vi "sCRIPT Bckup.vi"   [LabVIEW 2020]
uses:
  <userlib>/_OpenG.lib/lvzip/lvzip.llb/ZLIB Open ZIP Mode__ogtk.ctl
  <vilib>/addons/database/Connection.llb/Conn Execute.vi
  <vilib>/addons/database/Recordset.llb/Rec Fetch Recordset Data (R).vi
  <vilib>/addons/database/Recordset.llb/Rec Destroy - Connection.vi
  MS SQL/MS_Global.vi
  <vilib>/addons/database/NI_Database_API.lvlib
types:
  T1 = typedef "ZLIB Open ZIP Mode__ogtk.ctl" = enum16{"create new", "append to end", "append to archive"}
  T2 = typedef "TD SQL.ctl" = cluster{"MS SQL Connection":T3, "UDL File":path, "Time":string, "DCODE":string, "WIP+1":i64, "MC No?":i32, "POKAYOKE?":bool, "Expected Result":string, "Result [Status]":string, "Clock":dbl, "RFID":string, "WIP Queue":refnum<queue>, "TS Parameter":T4, "Data_Queue":refnum<queue>[], "RFID Serial No.":string}
  T3 = typedef "NI_Database_API.lvlib/Conn ObjectReference.ctl" = refnum<k1>
  T4 = typedef "TS_Parameter.ctl" = cluster{"ProfitCenterCode":string, "LineCode":string, "WorkOrderNumber":string, "Model":string, "Model_with_Prefix":string, "VendorCode":string, "SetParameterDateCode":string, "PokaYoke":i32, "Target":i32, "Live_DateCode":string, "CustomerPartNumber":string, "Hand":string, "sBarcode":bool, "FCA":i32, "Ent_Stamp":timestamp, "STS_CD":dbl}
  T5 = cluster{"Data Path":path, "Calibration Path":path, "Settings Path":path, "Script Path":path, "DAQ Support":path, "Reporting Desktop":path, "Help":path}
  T6 = typedef "NI_Database_API.lvlib/Rec ObjectReference.ctl" = refnum<k1>
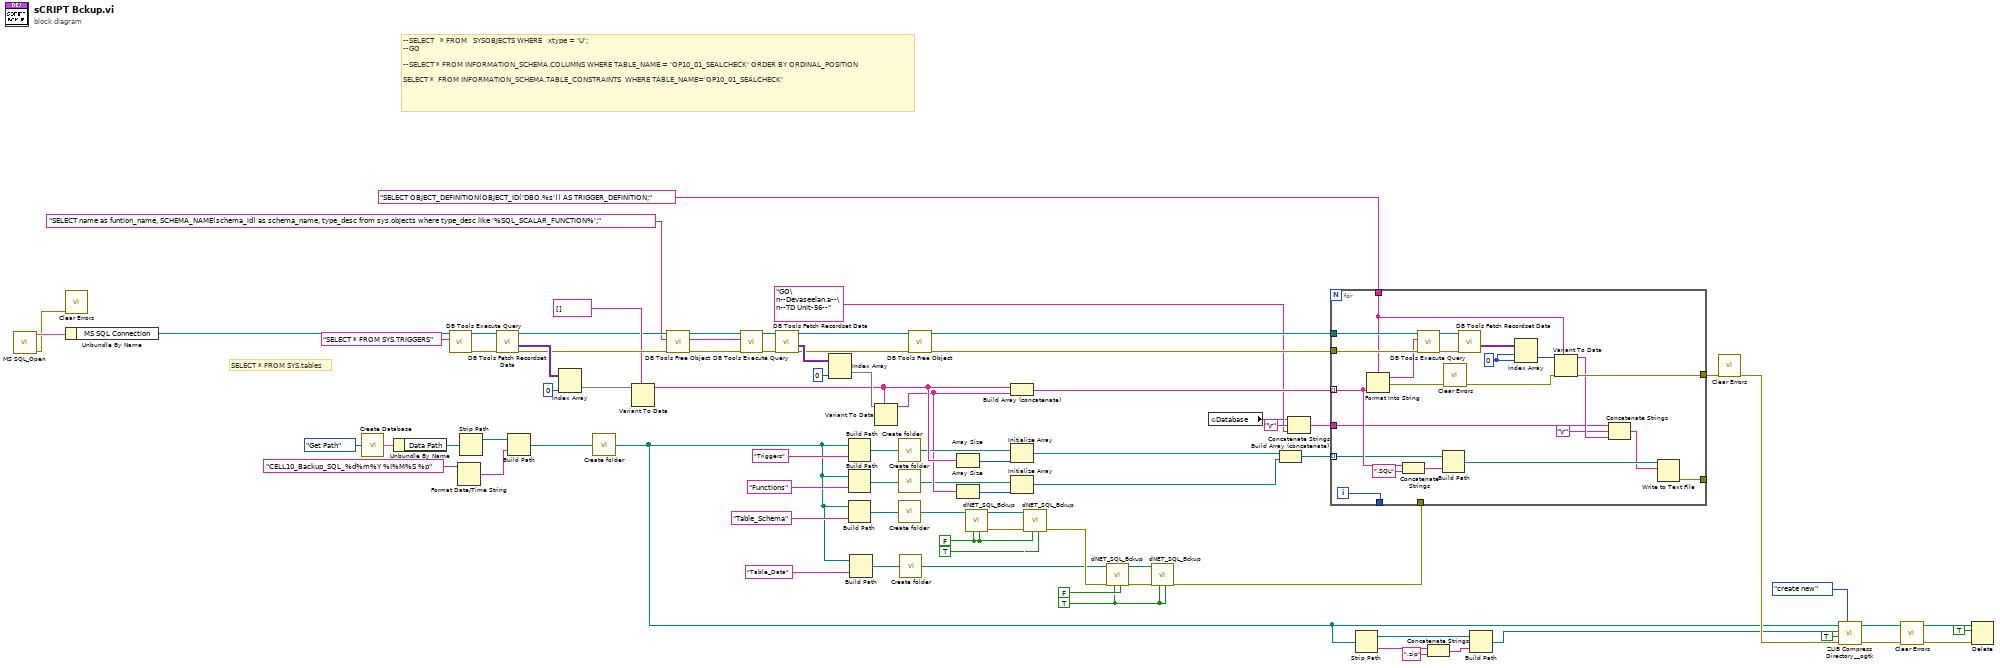
[diagram p0: block diagram]
diagram:
  w2 = TRUE ("Table Data")
  w8 = FALSE ("Table Data")
  # "--SELECT   * FROM   SYSOBJECTS WHERE   xtype = 'U';\n--GO\n\n--SELECT * FROM INFORMATION_SCHEMA.COLUMNS WHERE TABLE_NAME = 'OP10_01_SEALCHECK' ORDER BY ORDINAL_POSITION\n\nSELECT *  FROM INFORMATION_SCHEMA.TABLE_CONSTRAINTS  WHERE TABLE_NAME='OP10_01_SEALCHECK'"
  # "SELECT * FROM SYS.tables"
  n1 = call "MS SQL_Open.vi"() -> ("error out"=w28:errorcluster, "Ref Out"=w78:T2)  [unwired: 9 in, 1 out]
  n2 = call <vilib>:"Clear Errors.vi"("error in (no error)"=w28) -> ()  [unwired: 5 in, 2 out]
  n3 = Unbundle By Name(w78) -> ("MS SQL Connection"=w77:T3)
  n4 = call <userlib>:"Create Database.vi"("Get/Create"=enum16{"Get Path", "Create Path"}."Get Path") -> ("Path Out"=w35:T5)  [unwired: 13 in, 1 out]
  n5 = Unbundle By Name(w35) -> ("Data Path"=w34:path)
  n6 = call-poly <vilib>:"DB Tools Execute Query.vi"("SQL query"="SELECT * FROM SYS.TRIGGERS", "connection reference"=w77) -> ("error out"=w75:errorcluster, "recordset reference"=w76:T6)  [unwired: 6 in]
  n7 = Format Date/Time String(time format string (%c)="CELL10_Backup_SQL_%d%m%Y %I%M%S %p") -> (date/time string=w65:string)  [unwired: 2 in]
  n8 = Strip Path(path=w34) -> (stripped path=w33:path)  [unwired: 1 out]
  n9 = call-poly <vilib>:"DB Tools Fetch Recordset Data.vi"("error in (no error)"=w75, "recordset reference"=w76) -> ("error out"=w70:errorcluster, "recordset data"=w73:variant[][], "recordset reference out"=w64:T6)  [unwired: 3 in]
  n10 = Build Path(base path=w33, name or relative path=w65) -> (appended path=w66:path)
  n11 = Index Array(array=w73, index (col)=0 ("disabled index (col)")) -> (element=w71:variant[])  [unwired: 1 in]
  n12 = call <userlib>:"Create folder.vi"("Path In"=w66) -> ("Path out"=w11:path)  [unwired: 14 in]
  n13 = Variant To Data(type=string[] [], Variant=w71) -> (data=w52:string[])  [unwired: 1 in, 1 out]
  n14 = call-poly <vilib>:"DB Tools Free Object.vi"("error in (no error)"=w70, "recordset reference"=w64) -> ("error out"=w42:errorcluster, "connection reference"=w43:T3)  [unwired: 8 in]
  n15 = call-poly <vilib>:"DB Tools Execute Query.vi"("error in (no error)"=w42, "SQL query"="SELECT name as funtion_name, SCHEMA_NAME(schema_id) as schema_name, type_desc from sys.objects where type_desc like '%SQL_SCALAR_FUNCTION%';", "connection reference"=w43) -> ("error out"=w61:errorcluster, "recordset reference"=w62:T6)  [unwired: 5 in]
  n16 = call-poly <vilib>:"DB Tools Fetch Recordset Data.vi"("error in (no error)"=w61, "recordset reference"=w62) -> ("error out"=w41:errorcluster, "recordset data"=w59:variant[][], "recordset reference out"=w39:T6)  [unwired: 3 in]
  n17 = Index Array(array=w59, index (col)=0 ("disabled index (col)")) -> (element=w58:variant[])  [unwired: 1 in]
  n18 = Build Path(base path=w11, name or relative path="Triggers" ("time format string (%c)")) -> (appended path=w54:path)
  n19 = Build Path(base path=w11, name or relative path="Functions" ("time format string (%c)")) -> (appended path=w53:path)
  n20 = Build Path(base path=w11, name or relative path="Table_Schema" ("time format string (%c)")) -> (appended path=w12:path)
  n21 = Build Path(base path=w11, name or relative path="Table_Data" ("time format string (%c)")) -> (appended path=w13:path)
  n22 = Variant To Data(type=w52, Variant=w58) -> (data=w49:string[])  [unwired: 1 in, 1 out]
  n23 = call <userlib>:"Create folder.vi"("Path In"=w54) -> ("Path out"=w50:path)  [unwired: 14 in]
  n24 = call <userlib>:"Create folder.vi"("Path In"=w53) -> ("Path out"=w47:path)  [unwired: 14 in]
  n25 = call <userlib>:"Create folder.vi"("Path In"=w12) -> ("Path out"=w10:path)  [unwired: 14 in]
  n26 = call <userlib>:"Create folder.vi"("Path In"=w13) -> ("Path out"=w4:path)  [unwired: 14 in]
  n27 = call-poly <vilib>:"DB Tools Free Object.vi"("error in (no error)"=w41, "recordset reference"=w39) -> ("error out"=w40:errorcluster, "connection reference"=w38:T3)  [unwired: 8 in]
  n28 = Array Size(array=w52) -> (size(s)=w51:i32)
  n29 = Array Size(array=w49) -> (size(s)=w48:i32)
  n30 = call "dNET_SQL_Bckup.vi"("Bckup_DB?"=w8, "Table Data"=w8, "Table_Schema"=w10) -> ("error out"=w7:errorcluster)  [unwired: 8 in]
  n31 = Build Array (concatenate)(w52, w49) -> (w57:string[])
  n32 = Initialize Array(w50, w51) -> (w46:path[])
  n33 = Initialize Array(w47, w48) -> (w45:path[])
  n34 = call "dNET_SQL_Bckup.vi"("Bckup_DB?"=TRUE, "Table Data"=w8, "error in (no error)"=w7, "Table_Schema"=w10) -> ("error out"=w6:errorcluster)  [unwired: 7 in]
  n35 = call "dNET_SQL_Bckup.vi"("Bckup_DB?"=FALSE, "Table Data"=w2, "error in (no error)"=w6, "Table_Schema"=w4) -> ("error out"=w3:errorcluster)  [unwired: 7 in]
  n36 = call "dNET_SQL_Bckup.vi"("Bckup_DB?"=w2, "Table Data"=w2, "error in (no error)"=w3, "Table_Schema"=w4) -> ("error out"=w1:errorcluster)  [unwired: 7 in]
  n37 = global read "MS_Global.vi" "Database"() -> (w30:string)
  n38 = Build Array (concatenate)(w46, w45) -> (w44:path[])
  n39 = Concatenate Strings(w30, "\r", "GO\n--Devaseelan.a--\n--TD Unit-56--" ("string")) -> (w29:string)
  n40 = for {
    tunnel: w38 -> [w100]
    tunnel: w40 -> [w99]
    tunnel: "SELECT OBJECT_DEFINITION(OBJECT_ID('DBO.%s')) AS TRIGGER_DEFINITION;" ("SQL query") -> [w94]
    tunnel: w57 -> [w92] mode=indexing
    tunnel: [w93] -> w27
    tunnel: [w87] -> _
    tunnel: w44 -> [w85] mode=indexing
    tunnel: w29 -> [w81]
    tunnel: [w79] -> _
    tunnel: w1 -> [_]
    i -> [w79]
    w95 = 0 ("disabled index (col)")
    n41 = Format Into String(format string=w94, w92) -> (resulting string=w86:string, error out=w84:errorcluster)  [unwired: 2 in]
    n42 = Concatenate Strings(w92, ".SQL" ("string")) -> (w90:string)
    n43 = call-poly <vilib>:"DB Tools Execute Query.vi"("error in (no error)"=w99, "SQL query"=w86, "connection reference"=w100) -> ("error out"=w101:errorcluster, "recordset reference"=w98:T6)  [unwired: 5 in]
    n44 = Build Path(base path=w85, name or relative path=w90) -> (appended path=w89:path)
    n45 = call <vilib>:"Clear Errors.vi"("error in (no error)"=w84) -> ("error out"=w83:errorcluster)  [unwired: 5 in, 1 out]
    n46 = call-poly <vilib>:"DB Tools Fetch Recordset Data.vi"("error in (no error)"=w101, "recordset reference"=w98) -> ("recordset data"=w97:variant[][])  [unwired: 3 in, 2 out]
    n47 = Index Array(array=w97, index (row)=w95, index (col)=w95) -> (element=w96:variant)
    n48 = Variant To Data(error in=w83, type=w94, Variant=w96) -> (data=w88:string, error out=w93:errorcluster)
    n49 = Concatenate Strings(w81, "\r", w88) -> (w82:string)
    n50 = Write to Text File(file (use dialog)=w89, text=w82) -> (error out=w87:errorcluster)  [unwired: 2 in, 2 out]
  }
  n51 = Strip Path(path=w11) -> (stripped path=w25:path, name=w24:string)
  n52 = Concatenate Strings(w24, ".zip" ("string")) -> (w23:string)
  n53 = Build Path(base path=w25, name or relative path=w23) -> (appended path=w21:path)
  n54 = call <vilib>:"Clear Errors.vi"("error in (no error)"=w27) -> ("error out"=w26:errorcluster)  [unwired: 5 in, 1 out]
  n55 = call <userlib>:"ZLIB Compress Directory__ogtk.vi"("append (create new)"=ZLIB_Open_ZIP_Mode__ogtk."create new", "error in (no error)"=w26, "include subdirectories (F)"=TRUE, "archive name (root directory with .zip ending)"=w21, "root directory (file dialog)"=w11) -> ("error out"=w18:errorcluster, "root directory out"=w17:path)  [unwired: 4 in, 1 out]
  n56 = call <vilib>:"Clear Errors.vi"("error in (no error)"=w18) -> ("error out"=w16:errorcluster)  [unwired: 5 in, 1 out]
  n57 = Delete(path (use dialog)=w17, entire hierarchy (F)=TRUE, error in=w16) -> ()  [unwired: 2 in, 3 out]
